vi "Create HTTPS Server.vi"(8 "error in (no error)":errorcluster, 9 "Port":u16=443, 11 "Server in":refnum<class "Server.lvclass">) -> (0 "error out":errorcluster, 3 "Server out":refnum<class "Server.lvclass">)   [LabVIEW 2020, in "HTTP Server.lvlib" / "Server.lvclass"]
uses:
  Server.lvclass
  Server.lvclass/Server.ctl
  HTTP TCP Server/HTTP TCP Server.lvclass
  HTTPS Connection Callback.vi
  lv-stream/stream/Endpoint/Endpoint.lvclass
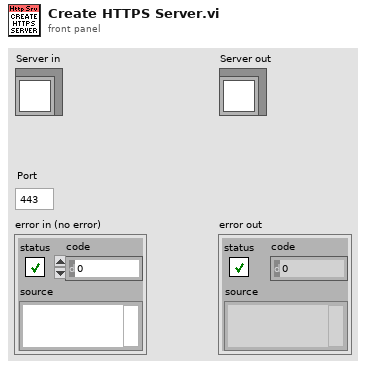
[diagram p1: front panel]
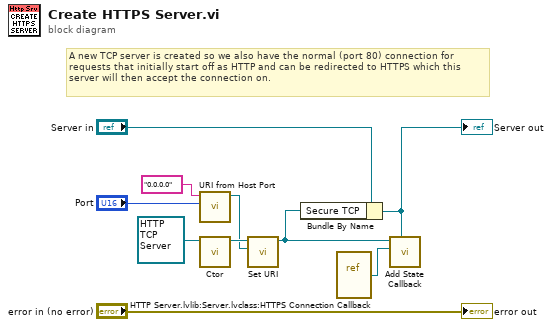
[diagram p0: block diagram]
diagram:
  # "A new TCP server is created so we also have the normal (port 80) connection for requests that initially start off as HTTP and can be redirected to HTTPS which this server will then accept the connection on."
  n1 = call "URI from Host Port.vi"("Port"="Port", "Host"="0.0.0.0") -> ("URI"=w8:refnum<class "URI.lvclass">)  [unwired: 9 in]
  n2 = call-dynamic "Ctor.vi"("TCP Server in"=refnum<class "HTTP TCP Server.lvclass"> refnum ("HTTP Server:HTTP TCP Server")) -> ("TCP Server out"=w9:refnum<class "HTTP TCP Server.lvclass">)  [unwired: 9 in, 1 out]
  n3 = call "Set URI.vi"("URI"=w8, "Endpoint in"=w9) -> ("Endpoint out"=w7:refnum<class "Endpoint.lvclass">)  [unwired: 8 in, 1 out]
  n4 = Bundle By Name(cluster="Server in", "Secure TCP"=w7) -> (w3:refnum<class "Server.lvclass">)
  "Server out" <- w3
  n5 = vi-ref "HTTP Server.lvlib:Server.lvclass:HTTPS Connection Callback.vi"() -> (w6:refnum<vi>)
  n6 = call-dynamic "Add State Callback.vi"("Owner (None)"=w3, "Callback"=w6, "Endpoint in"=w7) -> ()  [unwired: 7 in, 2 out]
  "error out" <- "error in (no error)"
